vi "Uses SubVI from LV Analysis Library.vi"() -> (0 "error out":errorcluster, 3 "signal out":waveform(dbl))   [LabVIEW 2012]
uses:
  <vilib>/measure/NI_MABase.lvlib
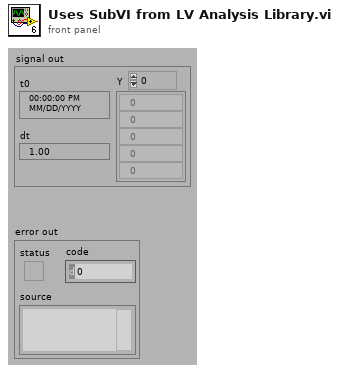
[diagram p1: front panel]
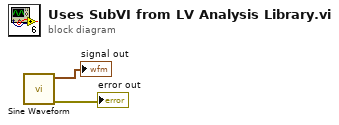
[diagram p0: block diagram]
diagram:
  n1 = call <vilib>:"Sine Waveform.vi"() -> ("error out"=→"error out":errorcluster, "signal out"=→"signal out":waveform(dbl))  [unwired: 7 in, 3 out]
